vi "UI.vi"(8 "error":errorcluster, 11 "2-axis":refnum<class "Syncronus 2-Axis Stage.lvclass">) -> (0 "error out":errorcluster)   [LabVIEW 2022 SP3, in "Controls.lvlib"]
uses:
  View/Controls.lvlib
  Syncronus 2-Axis Stage/Syncronus 2-Axis Stage.lvclass
panel:
  out "XY Position Graph":cluster{"X":dbl, "Y":dbl}[](graph)
  in  "Clear Error":bool
  in  "Set X-Speed":u16
  in  "Set Y-Speed":u16
  in  "Set X-Acceleration":u16
  in  "Set Y-Acceleration":u16
  out "X-Speed":dbl
  out "Y-Speed":dbl
  out "X-Current Speed":dbl
  out "Y-Current Speed":dbl
  out "X-Acceleration":dbl
  out "Y-Acceleration":dbl
  out "Y-Homed":bool
  out "X-Homed":bool
  out "X-Moving":bool
  out "Y-Moving":bool
  out "Y-Position":dbl
  out "X-Position":dbl
  out "Stage Error":errorcluster
  in  "Abort Motion":bool
  in  "Home Stage":bool
  in  "Move Stage":bool
  in  "Y-Destination":dbl
  in  "X-Destination":dbl
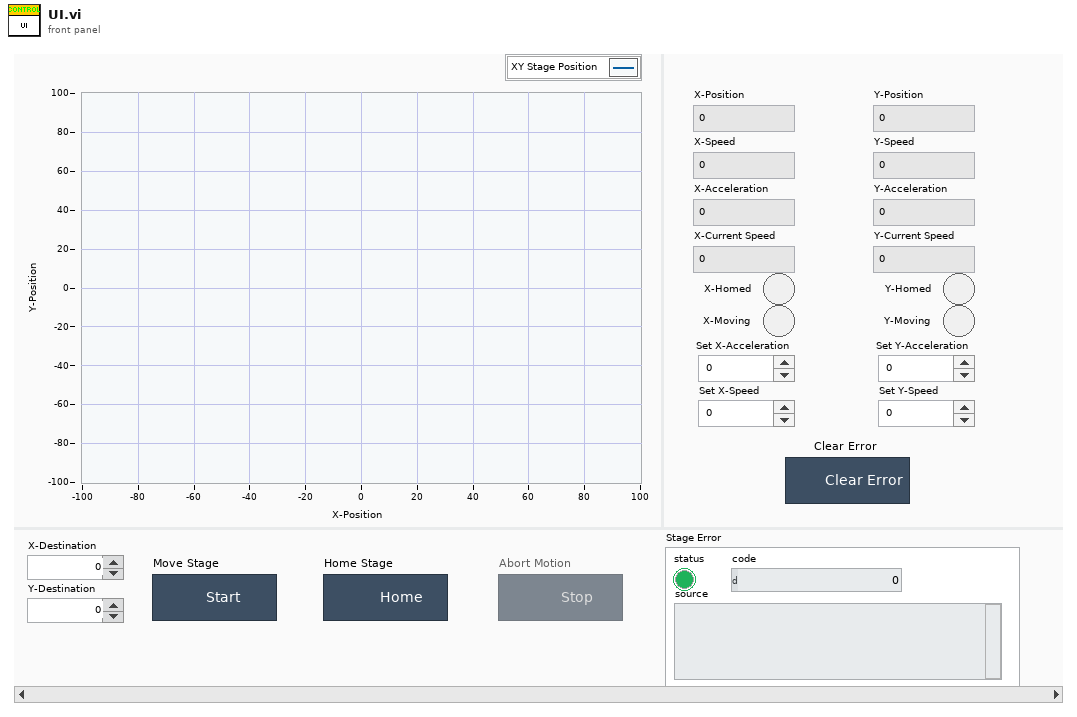
[diagram p1: front panel]
types:
  T1 = enum32{"Invalid", "Standard", "Closed", "Hidden", "Minimized", "Maximized"}
  T2 = enum32{"invalid app kind", "Development System", "Run Time System", "Student Edition", "Embedded LabVIEW", "Evaluation", "Custom"}
  T3 = enum8{"Enabled", "Disabled", "Disabled and Grayed Out"}
  T4 = cluster{"Core":cluster{"Current VI Reference":refnum<vi>, "Close Panel on Exit?":bool}, "2-axis":refnum<class "Syncronus 2-Axis Stage.lvclass">}
  T5 = cluster{"Current VI Reference":refnum<vi>, "Close Panel on Exit?":bool}
  T6 = cluster{"Current Position X":dbl, "Current Position Y":dbl}[]
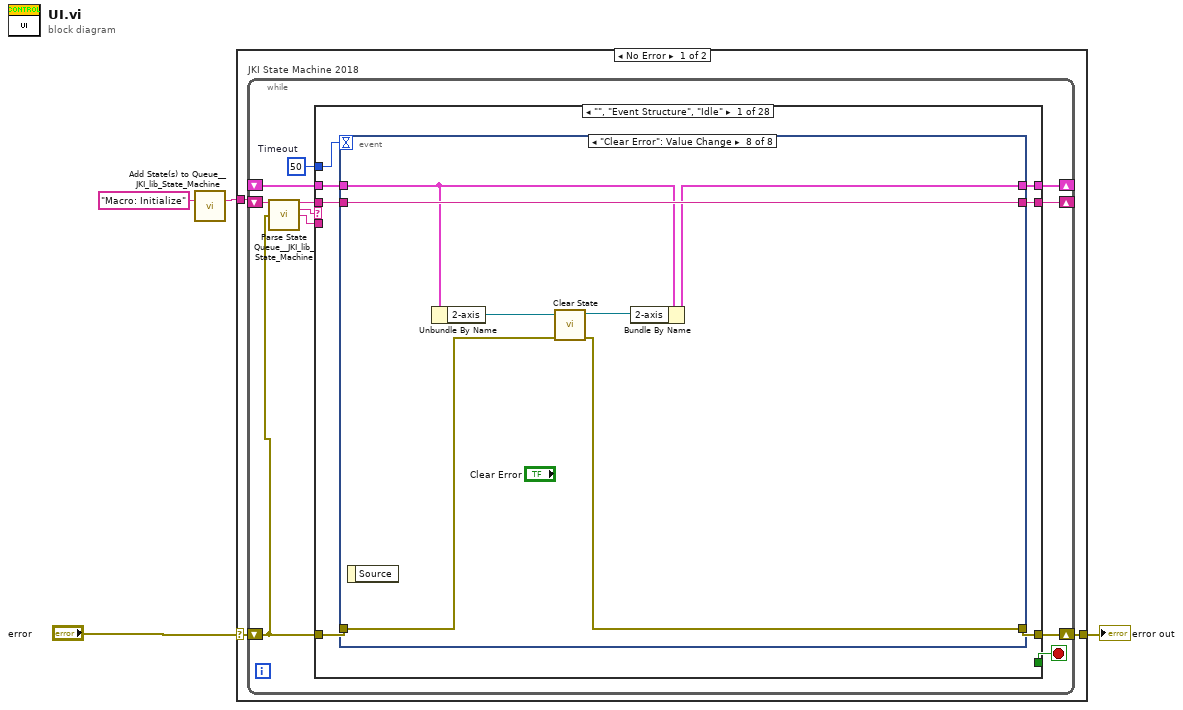
[diagram p0: block diagram]
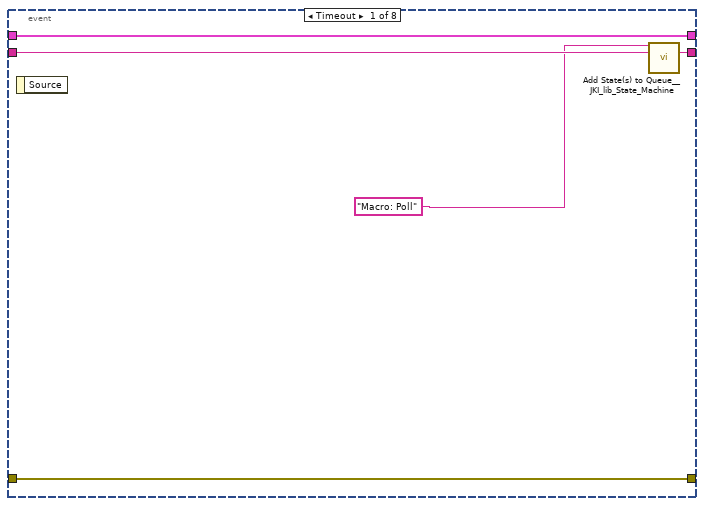
[diagram p2: hidden frame]
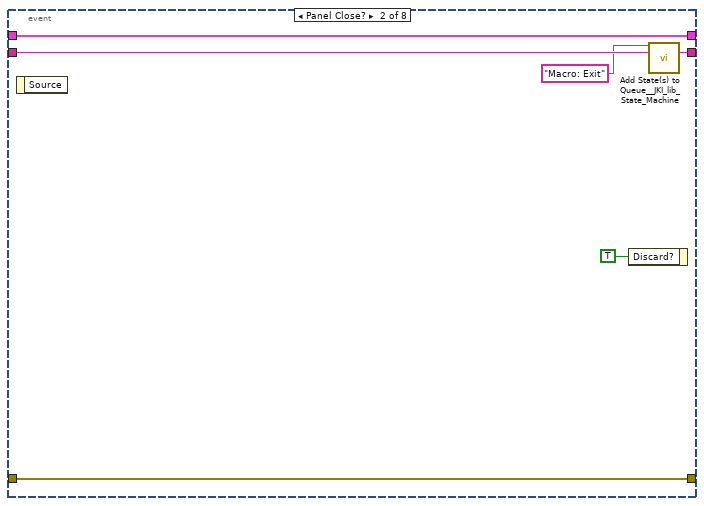
[diagram p3: hidden frame]
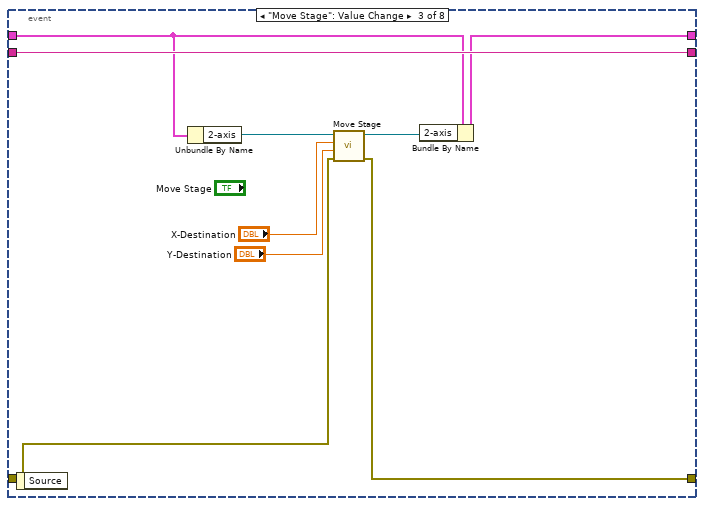
[diagram p4: hidden frame]
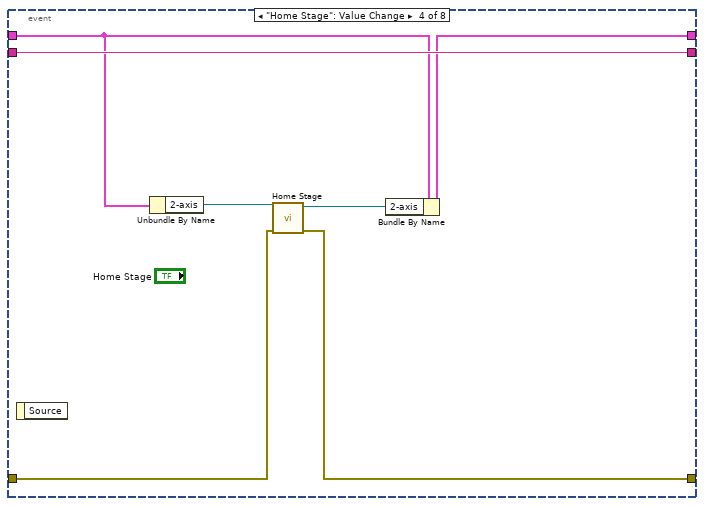
[diagram p5: hidden frame]
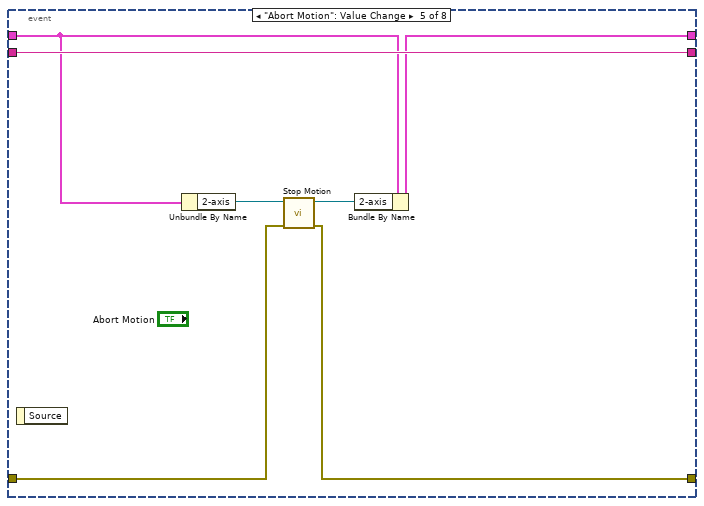
[diagram p6: hidden frame]
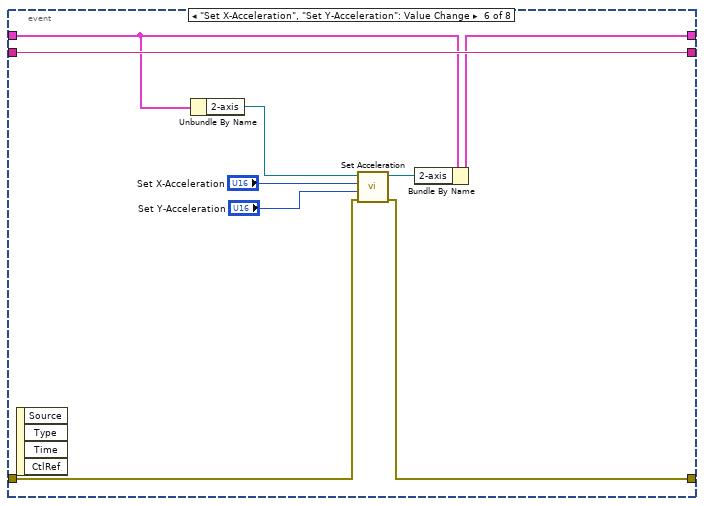
[diagram p7: hidden frame]
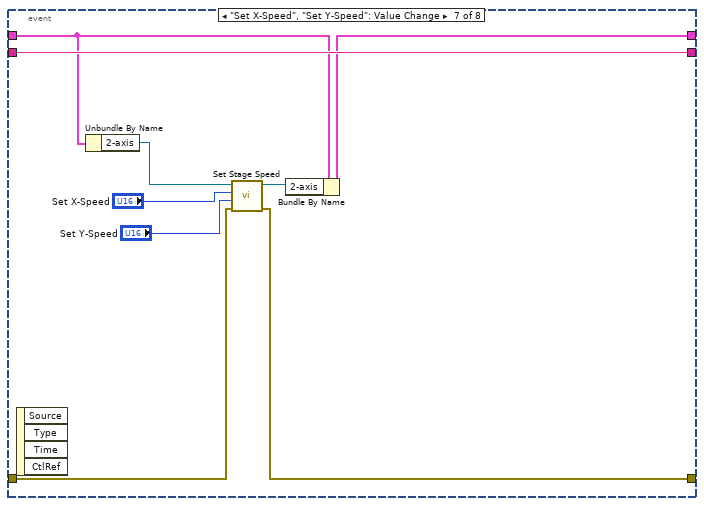
[diagram p8: hidden frame]
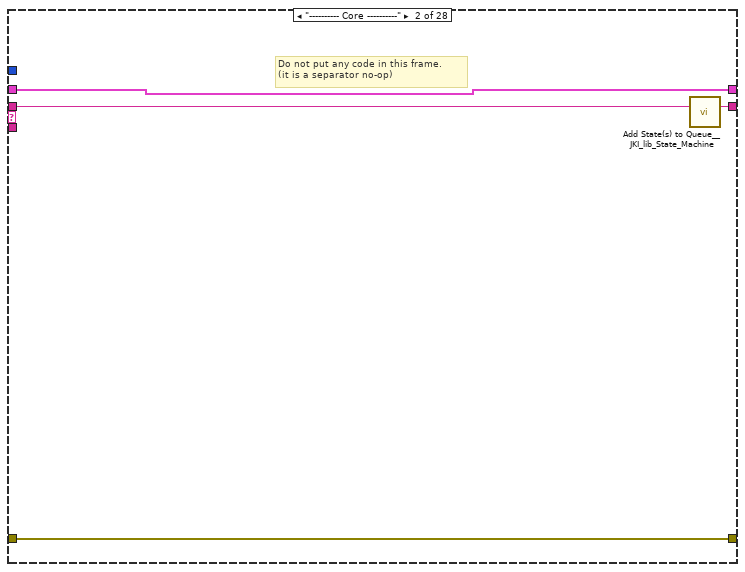
[diagram p9: hidden frame]
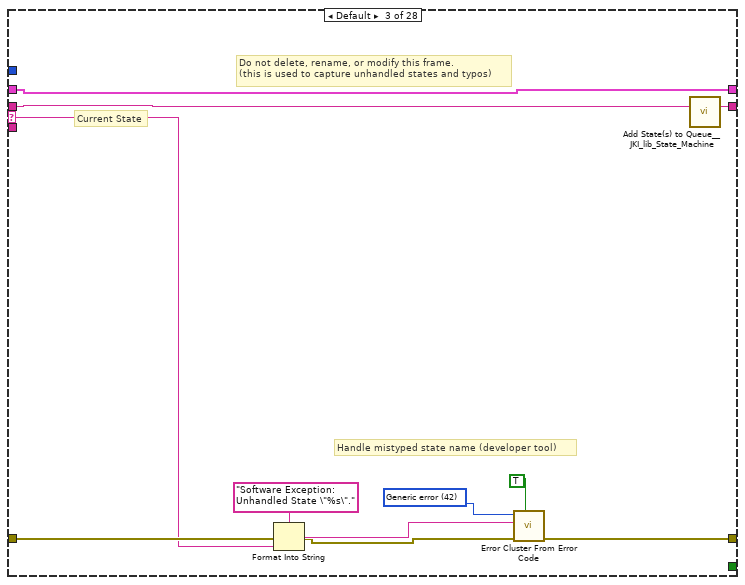
[diagram p10: hidden frame]
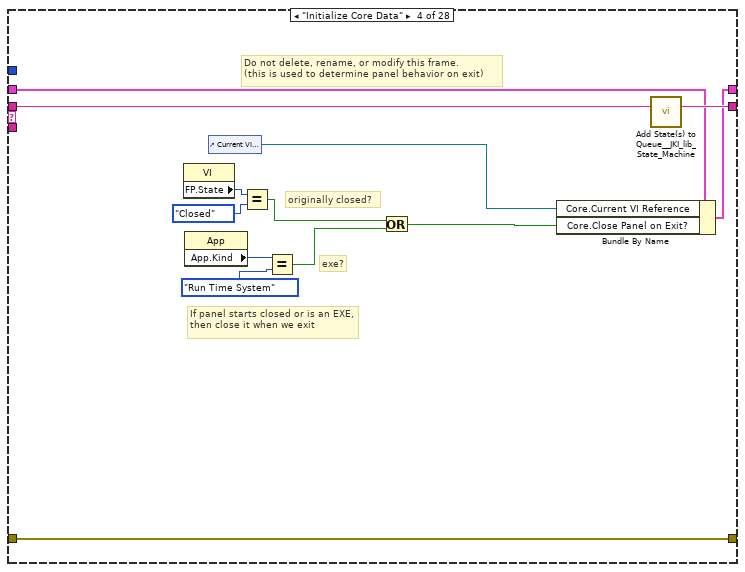
[diagram p11: hidden frame]
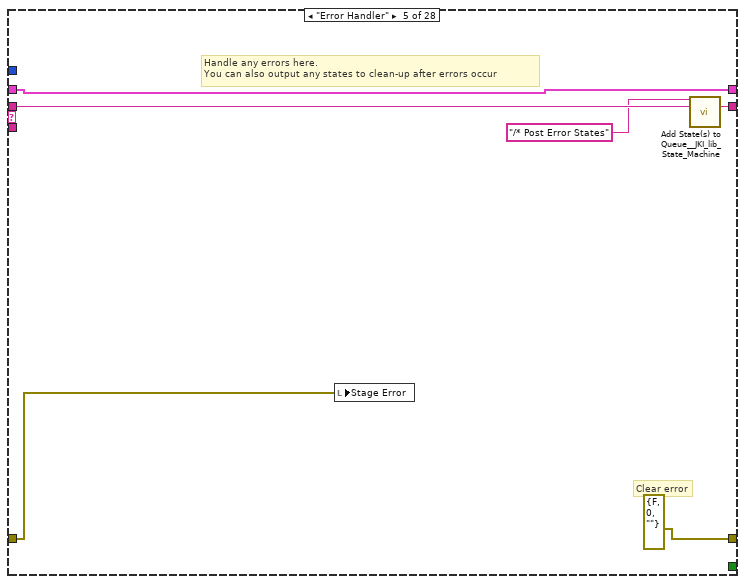
[diagram p12: hidden frame]
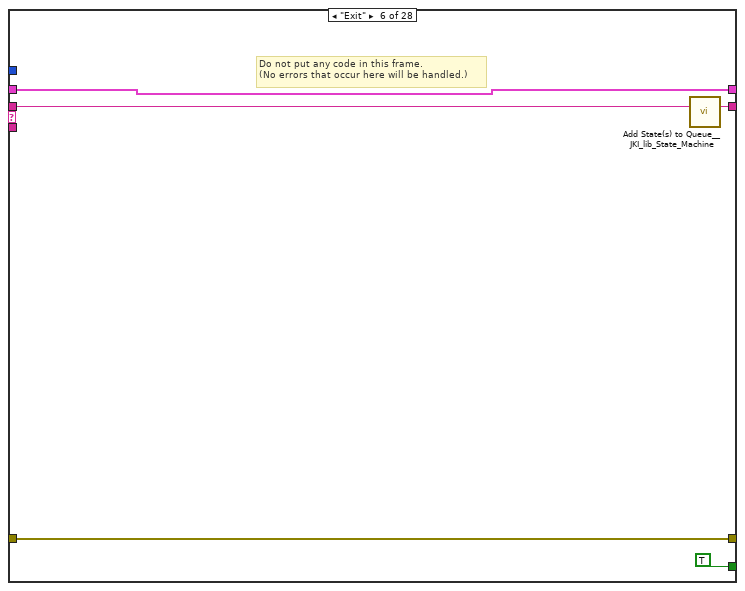
[diagram p13: hidden frame]
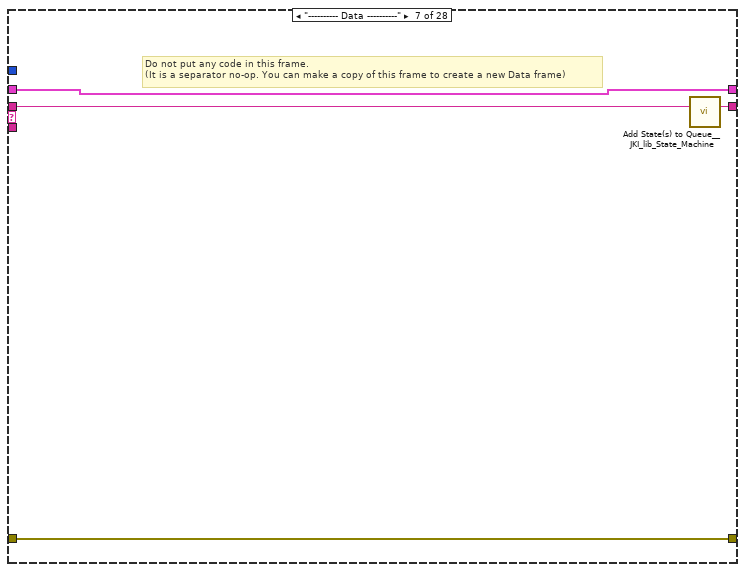
[diagram p14: hidden frame]
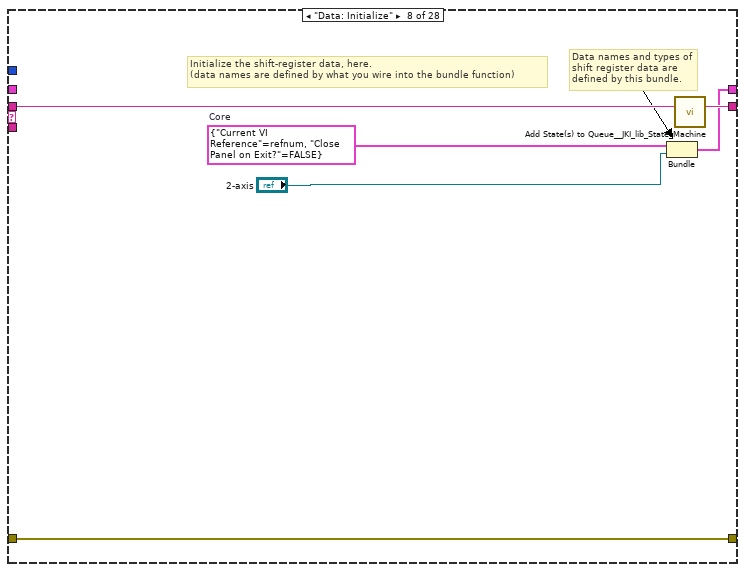
[diagram p15: hidden frame]
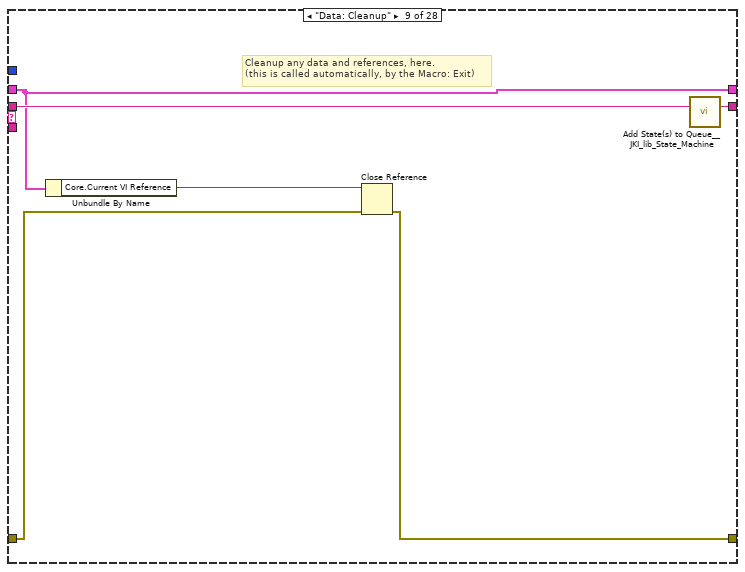
[diagram p16: hidden frame]
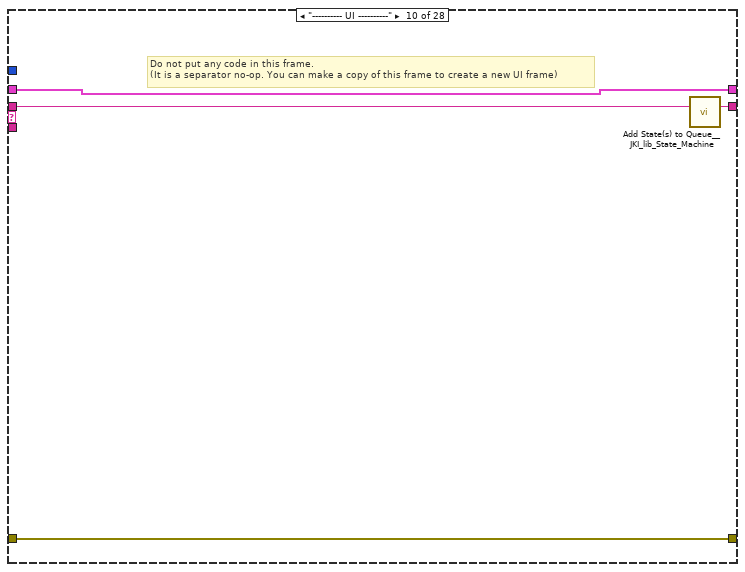
[diagram p17: hidden frame]
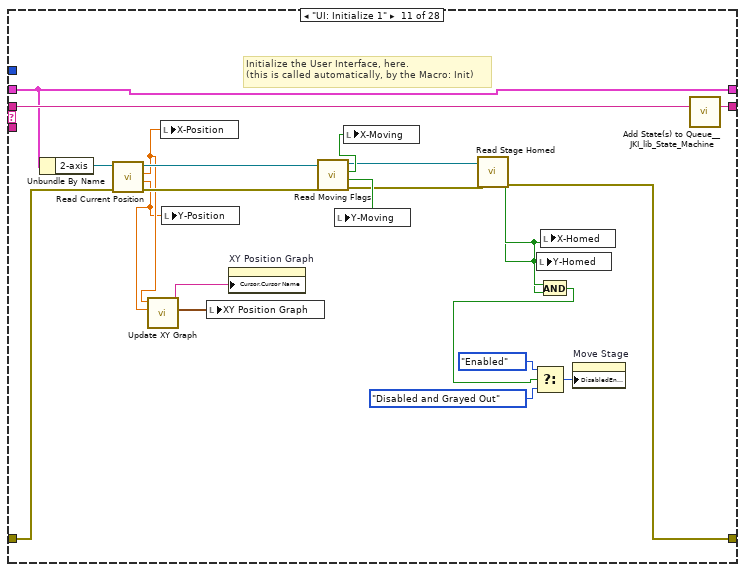
[diagram p18: hidden frame]
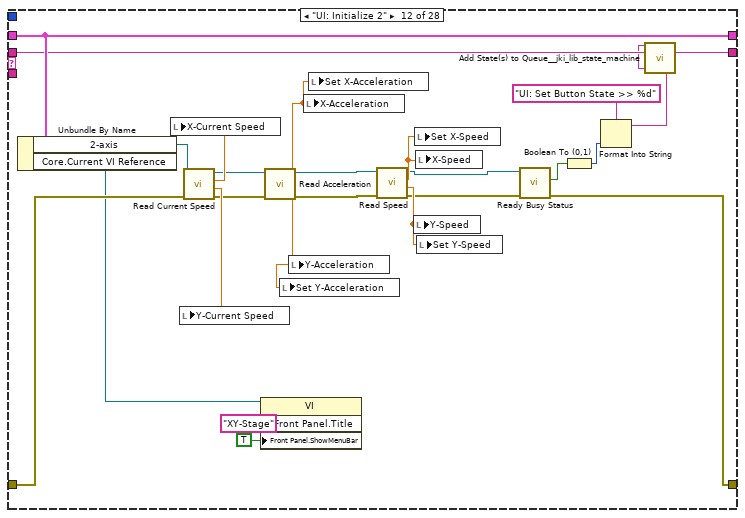
[diagram p19: hidden frame]
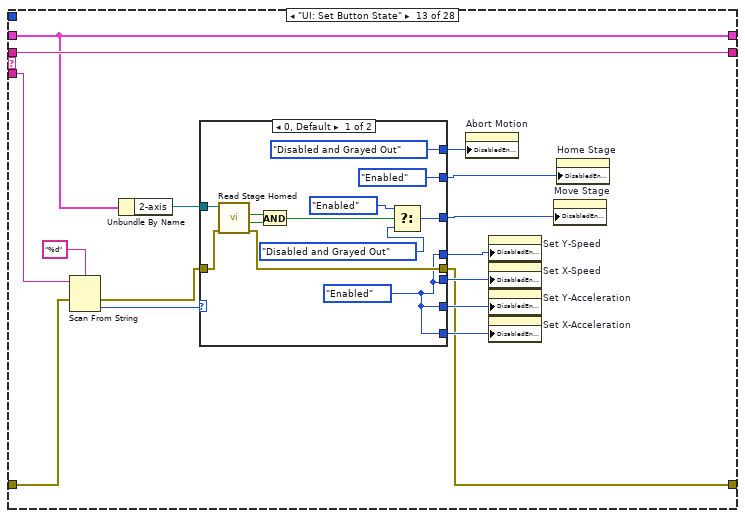
[diagram p20: hidden frame]
diagram:
  n1 = call <vilib>:"Add State(s) to Queue__JKI_lib_State_Machine.vi"("State(s) in (\"\")"="Macro: Initialize") -> ("States Out"=w1:string)  [unwired: 14 in]
  n2 = case shown="No Error" "error" {
    selector: "error" -> [w7 _]
    tunnel: [w6 _] -> w3
    tunnel: w1 -> [w5 _]
    frame No Error {
      n3 = while "JKI State Machine 2018" {
        shift-right: [w11] -> _
        shift-left: _ -> [w10]
        shift-right: [w14] -> w6
        shift-left: w7 -> [w8]
        shift-right: [w13] -> _
        shift-left: w5 -> [w15]
        stop <- w12 stop-if-true
        w9 = 50  # Timeout
        n4 = call <vilib>:"Parse State Queue__JKI_lib_State_Machine.vi"("State Queue"=w15, "Error In (no error)"=w8) -> ("Remaining States"=w17:string, "Current State"=w18:string, "Arguments"=w16:string)  [unwired: 11 in]
        n5 = case shown="\"\", \"Event Structure\", \"Idle\"" w18 {
          selector: w18 -> [_ _ w89 _ _ _ _ _ _ _ _ _ _ _ _ _ _ _ _ _ _ _ _ _ _ _ _ _]
          tunnel: w17 -> [w25 w88 w93 w112 w118 w123 w127 w133 w139 w143 w165 w177 w206 w227 w238 w307 w312 w322 w325 w330 w342 w351 w360 w369 w378 w384 w399 w407]
          tunnel: w16 -> [_ _ _ _ _ _ _ _ _ _ _ _ w196 w222 w232 _ _ _ _ _ _ _ _ _ _ _ _ _]
          tunnel: w10 -> [w23 w85 w91 w105 w115 w121 w124 _ w134 w140 w163 w180 w198 w225 w234 w304 w309 w319 w327 w329 w339 w350 w359 w368 w377 w388 w398 w406]
          tunnel: [w22 w86 w95 w109 errorcluster {"status"=FALSE, "code"=0, "source"=""} ("error out") w120 w125 w130 w135 w141 w149 w172 w193 w223 w235 w305 w310 w320 w323 w328 w333 w345 w354 w363 w372 w381 w395 w402] -> w14
          tunnel: w8 -> [w21 w86 w94 w109 w113 w120 w125 w130 w136 w141 w156 w179 w192 w224 w236 w305 w310 w320 w323 w328 w335 w346 w355 w364 w373 w382 w396 w403]
          tunnel: [w24 w87 w92 w111 w117 w122 w126 w132 w138 w142 w164 w178 w206 w226 w237 w306 w311 w321 w326 w330 w342 w351 w360 w369 w378 w385 w399 w407] -> w13
          tunnel: [_ _ _ _ _ TRUE _ _ _ _ _ _ _ _ _ _ _ _ _ _ _ _ _ _ _ _ _ _] -> w12
          tunnel: [w20 w85 w91 w110 w115 w121 w124 w131 w134 w140 w163 w180 w198 w225 w234 w304 w309 w319 w327 w329 w332 w344 w353 w362 w371 w380 w392 w401] -> w11
          tunnel: w9 -> [w19 _ _ _ _ _ _ _ _ _ _ _ _ _ _ _ _ _ _ _ _ _ _ _ _ _ _ _]
          frame "", "Event Structure", "Idle" {
            n6 = event shown="[7] \"Clear Error\": Value Change" {
              selector: _ -> [_ _ _ _ _ _ _ _]
              dyn-events: _ -> [_ _ _ _ _ _ _ _]
              timeout: w19 -> [_ _ _ _ _ _ _ _]
              tunnel: w25 -> [w30 w36 w45 w52 w59 w68 w77 w84]
              tunnel: [w29 w35 w45 w52 w59 w68 w77 w84] -> w24
              tunnel: w23 -> [w27 w33 w44 w51 w58 w67 w76 w83]
              tunnel: [w28 w34 w40 w49 w57 w63 w74 w81] -> w22
              tunnel: w21 -> [w28 w34 w41 w50 w56 w64 w75 w82]
              tunnel: [w27 w33 w38 w47 w54 w61 w70 w79] -> w20
              event Timeout {
                n7 = event-data() -> ()  [unwired: 1 in, 1 out]
                n8 = call <vilib>:"Add State(s) to Queue__JKI_lib_State_Machine.vi"("State(s) in Front (\"\")"="Macro: Poll", "State(s) in (\"\")"=w30) -> ("States Out"=w29:string)  [unwired: 13 in]
              }
              event Panel Close? {
                n9 = event-data() -> ()  [unwired: 1 in, 1 out]
                n10 = event-data("Discard?"=TRUE) -> ()  [unwired: 1 in, 1 out]
                n11 = call <vilib>:"Add State(s) to Queue__JKI_lib_State_Machine.vi"("State(s) in Front (\"\")"="Macro: Exit", "State(s) in (\"\")"=w36) -> ("States Out"=w35:string)  [unwired: 13 in]
              }
              event "Move Stage": Value Change {
                n12 = event-data() -> ()  [unwired: 1 in, 1 out]
                n13 = Unbundle By Name(w44) -> ("2-axis"=w39:refnum<class "Syncronus 2-Axis Stage.lvclass">)
                n14 = call-dynamic "Move Stage.vi"("error in (no error)"=w41, "Y Axis"="Y-Destination", "X Axis"="X-Destination", "2-Axis Stage in"=w39) -> ("error out"=w40:errorcluster, "2-Axis Stage out"=w37:refnum<class "Syncronus 2-Axis Stage.lvclass">)  [unwired: 6 in]
                n15 = Bundle By Name(cluster=w44, "2-axis"=w37) -> (w38:T4)
              }
              event "Home Stage": Value Change {
                n16 = event-data() -> ()  [unwired: 1 in, 1 out]
                n17 = Unbundle By Name(w51) -> ("2-axis"=w48:refnum<class "Syncronus 2-Axis Stage.lvclass">)
                n18 = call-dynamic "Home Stage.vi"("error in (no error)"=w50, "2-Axis Stage in"=w48) -> ("error out"=w49:errorcluster, "2-Axis Stage out"=w46:refnum<class "Syncronus 2-Axis Stage.lvclass">)  [unwired: 8 in]
                n19 = Bundle By Name(cluster=w51, "2-axis"=w46) -> (w47:T4)
              }
              event "Abort Motion": Value Change {
                n20 = event-data() -> ()  [unwired: 1 in, 1 out]
                n21 = Unbundle By Name(w58) -> ("2-axis"=w55:refnum<class "Syncronus 2-Axis Stage.lvclass">)
                n22 = call-dynamic "Stop Motion.vi"("error in (no error)"=w56, "2-Axis Stage in"=w55) -> ("error out"=w57:errorcluster, "2-Axis Stage out"=w53:refnum<class "Syncronus 2-Axis Stage.lvclass">)  [unwired: 8 in]
                n23 = Bundle By Name(cluster=w58, "2-axis"=w53) -> (w54:T4)
              }
              event "Set X-Acceleration", "Set Y-Acceleration": Value Change {
                n24 = event-data() -> ()  [unwired: 1 in, 4 out]
                n25 = Unbundle By Name(w67) -> ("2-axis"=w62:refnum<class "Syncronus 2-Axis Stage.lvclass">)
                n26 = call-dynamic "Set Acceleration.vi"("error in (no error)"=w64, "Y Axis"="Set Y-Acceleration", "X Axis"="Set X-Acceleration", "2-Axis Stage in"=w62) -> ("error out"=w63:errorcluster, "2-Axis Stage out"=w60:refnum<class "Syncronus 2-Axis Stage.lvclass">)  [unwired: 6 in]
                n27 = Bundle By Name(cluster=w67, "2-axis"=w60) -> (w61:T4)
              }
              event "Set X-Speed", "Set Y-Speed": Value Change {
                n28 = event-data() -> ()  [unwired: 1 in, 4 out]
                n29 = Unbundle By Name(w76) -> ("2-axis"=w71:refnum<class "Syncronus 2-Axis Stage.lvclass">)
                n30 = call-dynamic "Set Stage Speed.vi"("error in (no error)"=w75, "Y Axis"="Set Y-Speed", "X Axis"="Set X-Speed", "2-Axis Stage in"=w71) -> ("error out"=w74:errorcluster, "2-Axis Stage out"=w69:refnum<class "Syncronus 2-Axis Stage.lvclass">)  [unwired: 6 in]
                n31 = Bundle By Name(cluster=w76, "2-axis"=w69) -> (w70:T4)
              }
              event "Clear Error": Value Change {
                n32 = event-data() -> ()  [unwired: 1 in, 1 out]
                n33 = Unbundle By Name(w83) -> ("2-axis"=w80:refnum<class "Syncronus 2-Axis Stage.lvclass">)
                n34 = call-dynamic "Clear State.vi"("error in (no error)"=w82, "2-Axis Stage Status in"=w80) -> ("error out"=w81:errorcluster, "2-Axis Stage Status out"=w78:refnum<class "Syncronus 2-Axis Stage.lvclass">)  [unwired: 8 in]
                n35 = Bundle By Name(cluster=w83, "2-axis"=w78) -> (w79:T4)
              }
            }
          }
          frame "---------- Core ----------" {
            # "Do not put any code in this frame.\n(it is a separator no-op)"
            n36 = call <vilib>:"Add State(s) to Queue__JKI_lib_State_Machine.vi"("State(s) in (\"\")"=w88) -> ("States Out"=w87:string)  [unwired: 14 in]
          }
          frame Default {
            w98 = 42 items=["No error", "Argument error", "Memory is full", "Out of zone", "End of file", "File already open", "Generic file I/O error", "File not found", "File permission error", "Disk is full", "Duplicate path", "Too many files open", "System feature not enabled", "Resource file not found", "Cannot add resource", "Resource not found", "Image not found", "Image memory error", "Pen does not exist", "Config type invalid", "Config token not found", "Config parse error", "Config memory error", "Bad external code format", "Bad external code offset", "External code not present", "Null window", "Destroy window error", "Null menu", "Print aborted", "Bad print record", "Print driver error", "Windows error during printing", "Memory error during printing", "Print dialog error", "Generic print error", "Invalid device refnum", "Device not found", "Device parameter error", "Device unit error", "Cannot open device", "Device call aborted", "Generic error", "Cancelled by user", "Object ID too low", "Object ID too high", "Object not in heap", "Unknown heap", "Unknown object (invalid DefProc)", "Unknown object (DefProc not in table)", "Message out of range", "Invalid (null) method", "Unknown message", "Manager call not supported", "Bad address", "Network operation in progress", "Network operation timed out", "Connection is busy", "Network attribute not supported", "Network error", "Address in use", "System out of memory", "Connection aborted", "Connection refused", "Not connected", "Already connected", "Connection closed", "Initialization error (interapplication manager)", "Bad occurrence", "Wait on unbound occurrence handler", "Occurrence queue overflow", "Datalog type conflict", "Unused", "Unrecognized type (interapplication manager)", "Memory corrupt", "Failed to make temporary DLL", "Old CIN version", "Drag socket not found", "Failed to load drop-object", "Failed to register OLE object", "Failed to release OLE object", "Format specifier type mismatch", "Unknown format specifier", "Too few format specifiers", "Too many format specifiers", "Scan failed", "Newer CIN version", "Error converting to variant", "Runtime menu error", "Password tampered", "Variant attribute not found", "Incompatible variant data type", "Event data is not available", "Event Store is not present", "Occurrence is not found", "Event Queue is not created", "Event info is not available", "Refnum passed is NULL", "Error retrieving Class GUID", "Error retrieving CoClass GUID", "Error retrieving TypeLib GUID.", "Bad built application magic bytes.", "Specific driver is different from the specific driver associated with the Logical Name.", "There is no session opened to the class driver.", "Max Error", "MAX - Error with config objects", "MAX - Error loading configuration", "MAX - Group not supported"]
            # "Current State"
            # "Do not delete, rename, or modify this frame.\n(this is used to capture unhandled states and typos)"
            # "Handle mistyped state name (developer tool)"
            n37 = Format Into String(format string="Software Exception: Unhandled State \"%s\"." ("message"), error in=w94, w89) -> (resulting string=w97:string, error out=w96:errorcluster)  [unwired: 1 in]
            n38 = call <vilib>:"Error Cluster From Error Code.vi"("show call chain? (False)"=TRUE, "error in (no error)"=w96, "error message (\"\")"=w97, "error code (0)"=w98) -> ("error out"=w95:errorcluster)  [unwired: 5 in]
            n39 = call <vilib>:"Add State(s) to Queue__JKI_lib_State_Machine.vi"("State(s) in (\"\")"=w93) -> ("States Out"=w92:string)  [unwired: 14 in]
          }
          frame "Initialize Core Data" {
            # "Do not delete, rename, or modify this frame.\n(this is used to determine panel behavior on exit)"
            # "originally closed?"
            # "exe?"
            # "If panel starts closed or is an EXE, then close it when we exit"
            n40 = property class="VI"() -> ("FP.State"=w102:T1)  [unwired: 2 in, 2 out]
            n41 = property class="App"() -> ("App.Kind"=w108:T2)  [unwired: 2 in, 2 out]
            n42 = control-ref of="Current VI Reference"() -> (w103:refnum<vi>)
            n43 = Equal?(x=w102, y=T1."Closed" ("Front Panel Window:State")) -> (x = y?=w100:bool)
            n44 = Equal?(x=w108, y=T2."Run Time System" ("Application:Kind")) -> (x = y?=w106:bool)
            n45 = Or(x=w100, y=w106) -> (x .or. y?=w104:bool)
            n46 = Bundle By Name(cluster=w105, "Core.Current VI Reference"=w103, "Core.Close Panel on Exit?"=w104) -> (w110:T4)
            n47 = call <vilib>:"Add State(s) to Queue__JKI_lib_State_Machine.vi"("State(s) in (\"\")"=w112) -> ("States Out"=w111:string)  [unwired: 14 in]
          }
          frame "Error Handler" {
            # "Handle any errors here.\nYou can also output any states to clean-up after errors occur"
            # "Clear error"
            n48 = local write "Stage Error"(w113) -> ()
            n49 = call <vilib>:"Add State(s) to Queue__JKI_lib_State_Machine.vi"("State(s) in Front (\"\")"="/* Post Error States", "State(s) in (\"\")"=w118) -> ("States Out"=w117:string)  [unwired: 13 in]
          }
          frame "Exit" {
            # "Do not put any code in this frame.\n(No errors that occur here will be handled.)"
            n50 = call <vilib>:"Add State(s) to Queue__JKI_lib_State_Machine.vi"("State(s) in (\"\")"=w123) -> ("States Out"=w122:string)  [unwired: 14 in]
          }
          frame "---------- Data ----------" {
            # "Do not put any code in this frame.\n(It is a separator no-op. You can make a copy of this frame to create a new Data frame)"
            n51 = call <vilib>:"Add State(s) to Queue__JKI_lib_State_Machine.vi"("State(s) in (\"\")"=w127) -> ("States Out"=w126:string)  [unwired: 14 in]
          }
          frame "Data: Initialize" {
            w129 = T5 {"Current VI Reference"=refnum, "Close Panel on Exit?"=FALSE}  # Core
            # "Data names and types of shift register data are defined by this bundle."
            # "Initialize the shift-register data, here.\n(data names are defined by what you wire into the bundle function)"
            n52 = Bundle("Core"=w129, "2-axis"="2-axis") -> (w131:T4)  [unwired: 1 in]
            n53 = call <vilib>:"Add State(s) to Queue__JKI_lib_State_Machine.vi"("State(s) in (\"\")"=w133) -> ("States Out"=w132:string)  [unwired: 14 in]
          }
          frame "Data: Cleanup" {
            # "Cleanup any data and references, here.\n(this is called automatically, by the Macro: Exit)"
            n54 = Unbundle By Name(w134) -> ("Core.Current VI Reference"=w137:refnum<vi>)
            n55 = Close Reference(reference=w137, error in (no error)=w136) -> (error out=w135:errorcluster)
            n56 = call <vilib>:"Add State(s) to Queue__JKI_lib_State_Machine.vi"("State(s) in (\"\")"=w139) -> ("States Out"=w138:string)  [unwired: 14 in]
          }
          frame "---------- UI ----------" {
            # "Do not put any code in this frame.\n(It is a separator no-op. You can make a copy of this frame to create a new UI frame)"
            n57 = call <vilib>:"Add State(s) to Queue__JKI_lib_State_Machine.vi"("State(s) in (\"\")"=w143) -> ("States Out"=w142:string)  [unwired: 14 in]
          }
          frame "UI: Initialize 1" {
            # "Initialize the User Interface, here.\n(this is called automatically, by the Macro: Init)"
            n58 = Unbundle By Name(w163) -> ("2-axis"=w144:refnum<class "Syncronus 2-Axis Stage.lvclass">)
            n59 = call-dynamic "Read Current Position.vi"("error in (no error)"=w156, "2-Axis Stage Status in"=w144) -> ("error out"=w158:errorcluster, "Y Position"=w147:dbl, "X Position"=w148:dbl, "2-Axis Stage Status out"=w160:refnum<class "Syncronus 2-Axis Stage.lvclass">)  [unwired: 6 in]
            n60 = call "Update XY Graph.vi"("Current Position Y"=w147, "Current Position X"=w148) -> ("Array"=w146:T6, "String"=w145:string)  [unwired: 7 in, 1 out]
            n61 = local write "X-Position"(w148) -> ()
            n62 = local write "Y-Position"(w147) -> ()
            n63 = local write "XY Position Graph"(w146) -> ()
            n64 = property on="XY Position Graph" class="XYGraph (strict)"("Cursor.Cursor Name"=w145) -> ()  [unwired: 2 in, 2 out]
            n65 = call-dynamic "Read Moving Flags.vi"("error in (no error)"=w158, "2-Axis Stage Status in"=w160) -> ("error out"=w157:errorcluster, "Y-Axis Moving"=w161:bool, "X-Axis Moving"=w162:bool, "2-Axis Stage Status out"=w159:refnum<class "Syncronus 2-Axis Stage.lvclass">)  [unwired: 6 in]
            n66 = local write "Y-Moving"(w161) -> ()
            n67 = local write "X-Moving"(w162) -> ()
            n68 = call-dynamic "Read Stage Homed.vi"("error in (no error)"=w157, "2-Axis Stage Status in"=w159) -> ("error out"=w149:errorcluster, "Y-Axis Homed Moving"=w154:bool, "X-Axis Homed"=w155:bool)  [unwired: 6 in, 1 out]
            n69 = local write "Y-Homed"(w154) -> ()
            n70 = And(x=w155, y=w154) -> (x .and. y?=w153:bool)
            n71 = Select(t=T3."Enabled" ("Disabled"), s=w153, f=T3."Disabled and Grayed Out" ("Disabled")) -> (s? t:f=w151:T3)
            n72 = local write "X-Homed"(w155) -> ()
            n73 = property on="Move Stage" class="Bool"("DisabledEnum"=w151) -> ()  [unwired: 2 in, 2 out]
            n74 = call <vilib>:"Add State(s) to Queue__JKI_lib_State_Machine.vi"("State(s) in (\"\")"=w165) -> ("States Out"=w164:string)  [unwired: 14 in]
          }
          frame "UI: Initialize 2" {
            n75 = Unbundle By Name(w180) -> ("2-axis"=w166:refnum<class "Syncronus 2-Axis Stage.lvclass">, "Core.Current VI Reference"=w169:refnum<vi>)
            n76 = call-dynamic "Read Current Speed.vi"("error in (no error)"=w179, "2-Axis Stage Status in"=w166) -> ("error out"=w187:errorcluster, "Y Current Speed"=w190:dbl, "X Current Speed"=w189:dbl, "2-Axis Stage Status out"=w188:refnum<class "Syncronus 2-Axis Stage.lvclass">)  [unwired: 6 in]
            n77 = local write "X-Current Speed"(w189) -> ()
            n78 = local write "Y-Current Speed"(w190) -> ()
            n79 = property class="VI"(reference=w169, "Front Panel.Title"="XY-Stage" ("Front Panel Window:Title"), "Front Panel.ShowMenuBar"=TRUE ("Front Panel Window:Show Menu Bar")) -> ()  [unwired: 1 in, 2 out]
            n80 = call-dynamic "Read Acceleration.vi"("error in (no error)"=w187, "2-Axis Stage Status in"=w188) -> ("error out"=w185:errorcluster, "Y Acceleration"=w181:dbl, "X Acceleration"=w182:dbl, "2-Axis Stage Status out"=w186:refnum<class "Syncronus 2-Axis Stage.lvclass">)  [unwired: 6 in]
            n81 = local write "Set Y-Acceleration"(w181) -> ()
            n82 = local write "Y-Acceleration"(w181) -> ()
            n83 = local write "X-Acceleration"(w182) -> ()
            n84 = local write "Set X-Acceleration"(w182) -> ()
            n85 = call-dynamic "Read Speed.vi"("error in (no error)"=w185, "2-Axis Stage Status in"=w186) -> ("error out"=w173:errorcluster, "Y-Axis Speed"=w183:dbl, "X-Axis Speed"=w184:dbl, "2-Axis Stage Status out"=w174:refnum<class "Syncronus 2-Axis Stage.lvclass">)  [unwired: 6 in]
            n86 = local write "Y-Speed"(w183) -> ()
            n87 = local write "Set X-Speed"(w184) -> ()
            n88 = local write "X-Speed"(w184) -> ()
            n89 = local write "Set Y-Speed"(w183) -> ()
            n90 = call-dynamic "Ready Busy Status.vi"("error in (no error)"=w173, "2-Axis Stage Status in"=w174) -> ("error out"=w172:errorcluster, "Busy"=w171:bool)  [unwired: 7 in, 1 out]
            n91 = Boolean To (0,1)(Boolean=w171) -> (0, 1=w170:i16)
            n92 = Format Into String(format string="UI: Set Button State >> %d", w170) -> (resulting string=w175:string)  [unwired: 2 in, 1 out]
            n93 = call <vilib>:"Add State(s) to Queue__jki_lib_state_machine.vi"("State(s) in Front (\"\")"=w175, "State(s) in (\"\")"=w177) -> ("States Out"=w178:string)  [unwired: 13 in]
          }
          frame "UI: Set Button State" {
            n94 = Scan From String(format string="%d", input string=w196, error in=w192) -> (error out=w191:errorcluster, output 1=w194:i32)  [unwired: 2 in, 2 out]
            n95 = Unbundle By Name(w198) -> ("2-axis"=w197:refnum<class "Syncronus 2-Axis Stage.lvclass">)
            n96 = case shown="0, Default" w194 {
              tunnel: [T3."Enabled" ("Disabled") w220] -> w205
              tunnel: [T3."Disabled and Grayed Out" ("Disabled") T3."Enabled" ("Disabled")] -> w204
              tunnel: [w211 w220] -> w203
              tunnel: [w210 w219] -> w193
              tunnel: [w209 w220] -> w202
              tunnel: [w209 w220] -> w201
              tunnel: [w209 w220] -> w200
              tunnel: [w209 w220] -> w199
              tunnel: w197 -> [w207 _]
              tunnel: w191 -> [w208 w219]
              frame 0, Default {
                w209 = T3."Enabled" ("Disabled")
                n97 = call-dynamic "Read Stage Homed.vi"("error in (no error)"=w208, "2-Axis Stage Status in"=w207) -> ("error out"=w210:errorcluster, "Y-Axis Homed Moving"=w215:bool, "X-Axis Homed"=w216:bool)  [unwired: 6 in, 1 out]
                n98 = And(x=w216, y=w215) -> (x .and. y?=w214:bool)
                n99 = Select(t=T3."Enabled" ("Disabled"), s=w214, f=T3."Disabled and Grayed Out" ("Disabled")) -> (s? t:f=w211:T3)
              }
              frame 1 {
                w220 = T3."Disabled and Grayed Out" ("Disabled")
              }
            }
            n100 = property on="Abort Motion" class="Bool"("DisabledEnum"=w204) -> ()  [unwired: 2 in, 2 out]
            n101 = property on="Set Y-Speed" class="DigNum (strict)"("DisabledEnum"=w202) -> ()  [unwired: 2 in, 2 out]
            n102 = property on="Set X-Speed" class="DigNum (strict)"("DisabledEnum"=w201) -> ()  [unwired: 2 in, 2 out]
            n103 = property on="Set Y-Acceleration" class="DigNum (strict)"("DisabledEnum"=w200) -> ()  [unwired: 2 in, 2 out]
            n104 = property on="Set X-Acceleration" class="DigNum (strict)"("DisabledEnum"=w199) -> ()  [unwired: 2 in, 2 out]
            n105 = property on="Move Stage" class="Bool"("DisabledEnum"=w203) -> ()  [unwired: 2 in, 2 out]
            n106 = property on="Home Stage" class="Bool"("DisabledEnum"=w205) -> ()  [unwired: 2 in, 2 out]
          }
          frame "UI: Cursor Set" {
            # "Argument"
            # "Set and Unset Cursor Busy.\n(Usage: \"UI: Cursor Set >> Busy|Idle\")"
            n107 = case shown="\"Idle\", Default" w222 {
              tunnel: w224 -> [w229 w231]
              tunnel: [w228 w230] -> w223
              frame "Idle", Default {
                n108 = call <vilib>:"Unset Busy.vi"("error in (no error)"=w229) -> ("error out"=w228:errorcluster)  [unwired: 10 in]
              }
              frame "Busy" {
                n109 = call <vilib>:"Set Busy.vi"("error in (no error)"=w231) -> ("error out"=w230:errorcluster)  [unwired: 9 in, 1 out]
              }
            }
            n110 = call <vilib>:"Add State(s) to Queue__JKI_lib_State_Machine.vi"("State(s) in (\"\")"=w227) -> ("States Out"=w226:string)  [unwired: 14 in]
          }
          frame "UI: Front Panel State" {
            # "Argument"
            # "Set Front Panel Open or Closed\n(Usage: \"UI: Front Panel State >> Open|Close\")"
            n111 = Unbundle By Name(w234) -> ("Core.Current VI Reference"=w233:refnum<vi>)
            n112 = case shown="\"Minimize\", \"Minimized\"" w232 {
              tunnel: w236 -> [w244 w259 w270 w283 w296]
              tunnel: [w246 w260 w272 w285 w298] -> w235
              tunnel: w233 -> [w245 w257 w271 w284 w297]
              frame "Open", "Standard", Default {
                w239 = T1."Standard" ("State")
                n113 = property class="VI"(reference=w245, error in=w244) -> (reference out=w242:refnum<vi>, error out=w243:errorcluster, "FP.State"=w241:T1)
                n114 = Not Equal?(x=w241, y=w239) -> (x != y?=w240:bool)
                n115 = case shown="True" w240 {
                  tunnel: [w250 w252] -> w246
                  tunnel: w243 -> [w249 w252]
                  tunnel: w242 -> [w248 _]
                  tunnel: w239 -> [w247 _]
                  frame True {
                    n116 = invoke class="VI" method="FP.Open"(reference=w248, error in=w249, "Activate"=TRUE, "State"=w247) -> (error out=w250:errorcluster)  [unwired: 1 in, 4 out]
                  }
                  frame False {
                  }
                }
              }
              frame "Close", "Closed" {
                n117 = property class="VI"(reference=w257, error in=w259) -> (reference out=w256:refnum<vi>, error out=w258:errorcluster, "FP.State"=w254:T1)
                n118 = Not Equal?(x=w254, y=T1."Closed" ("Front Panel Window:State")) -> (x != y?=w253:bool)
                n119 = case shown="True" w253 {
                  tunnel: [w261 w264] -> w260
                  tunnel: w258 -> [w261 w263]
                  tunnel: w256 -> [_ w262]
                  frame False {
                  }
                  frame True {
                    n120 = invoke class="VI" method="FP.Close"(reference=w262, error in=w263) -> (error out=w264:errorcluster)  [unwired: 1 in, 2 out]
                  }
                }
              }
              frame "Hidden", "Hide" {
                w265 = T1."Hidden" ("State")
                n121 = property class="VI"(reference=w271, error in=w270) -> (reference out=w268:refnum<vi>, error out=w269:errorcluster, "FP.State"=w267:T1)
                n122 = Not Equal?(x=w267, y=w265) -> (x != y?=w266:bool)
                n123 = case shown="True" w266 {
                  tunnel: [w276 w277] -> w272
                  tunnel: w269 -> [w275 w277]
                  tunnel: w268 -> [w274 _]
                  tunnel: w265 -> [w273 _]
                  frame True {
                    n124 = invoke class="VI" method="FP.Open"(reference=w274, error in=w275, "State"=w273) -> (error out=w276:errorcluster)  [unwired: 2 in, 4 out]
                  }
                  frame False {
                  }
                }
              }
              frame "Minimize", "Minimized" {
                w278 = T1."Minimized" ("State")
                n125 = property class="VI"(reference=w284, error in=w283) -> (reference out=w281:refnum<vi>, error out=w282:errorcluster, "FP.State"=w280:T1)
                n126 = Not Equal?(x=w280, y=w278) -> (x != y?=w279:bool)
                n127 = case shown="True" w279 {
                  tunnel: [w289 w290] -> w285
                  tunnel: w282 -> [w288 w290]
                  tunnel: w281 -> [w287 _]
                  tunnel: w278 -> [w286 _]
                  frame True {
                    n128 = invoke class="VI" method="FP.Open"(reference=w287, error in=w288, "State"=w286) -> (error out=w289:errorcluster)  [unwired: 2 in, 4 out]
                  }
                  frame False {
                  }
                }
              }
              frame "Maximize", "Maximized" {
                w291 = T1."Maximized" ("State")
                n129 = property class="VI"(reference=w297, error in=w296) -> (reference out=w294:refnum<vi>, error out=w295:errorcluster, "FP.State"=w293:T1)
                n130 = Not Equal?(x=w293, y=w291) -> (x != y?=w292:bool)
                n131 = case shown="True" w292 {
                  tunnel: [w302 w303] -> w298
                  tunnel: w295 -> [w301 w303]
                  tunnel: w294 -> [w300 _]
                  tunnel: w291 -> [w299 _]
                  frame True {
                    n132 = invoke class="VI" method="FP.Open"(reference=w300, error in=w301, "State"=w299) -> (error out=w302:errorcluster)  [unwired: 2 in, 4 out]
                  }
                  frame False {
                  }
                }
              }
            }
            n133 = call <vilib>:"Add State(s) to Queue__JKI_lib_State_Machine.vi"("State(s) in (\"\")"=w238) -> ("States Out"=w237:string)  [unwired: 14 in]
          }
          frame "---------- Macro ----------" {
            # "Do not put any code in this frame.\n(It is a separator no-op. You can make a copy of this frame to create a new Macro frame)"
            n134 = call <vilib>:"Add State(s) to Queue__JKI_lib_State_Machine.vi"("State(s) in (\"\")"=w307) -> ("States Out"=w306:string)  [unwired: 14 in]
          }
          frame "Macro: Initialize" {
            w308 = "Data: Initialize\nInitialize Core Data\nUI: Initialize 1\nUI: Initialize 2\nUI: Front Panel State >> Open"  # Data: Initialize Initialize Core Data UI: Initialize 1 UI: Initialize 2 UI: Front Panel State >> Open
            # "Initialization Macro\n(This is called once, when the VI starts)"
            n135 = call <vilib>:"Add State(s) to Queue__JKI_lib_State_Machine.vi"("State(s) in Front (\"\")"=w308, "State(s) in (\"\")"=w312) -> ("States Out"=w311:string)  [unwired: 13 in]
          }
          frame "Macro: Exit" {
            # "Exit Macro\n(This is called once, when the VI exits)"
            n136 = Unbundle By Name(w319) -> ("Core.Close Panel on Exit?"=w318:bool)
            n137 = Select(t="UI: Front Panel State >> Close", s=w318, f="") -> (s? t:f=w315:string)
            n138 = call <vilib>:"Add State(s) to Queue__JKI_lib_State_Machine.vi"("State(s) in (\"\")"=w315, "State(s) at Back (\"\")"="Data: Cleanup\nExit") -> ("States Out"=w313:string)  [unwired: 13 in]
            n139 = call <vilib>:"Add State(s) to Queue__JKI_lib_State_Machine.vi"("State(s) in Front (\"\")"=w313, "State(s) in (\"\")"=w322) -> ("States Out"=w321:string)  [unwired: 13 in]
          }
          frame "Macro: Poll" {
            n140 = call <vilib>:"Add State(s) to Queue__jki_lib_state_machine.vi"("State(s) in Front (\"\")"="Stage: Get Latest Position\nStage: Get Moving Status\nStage: Get Homed Status\nStage: Get Acceleration\nStage: Get Current Speed\nStage: Get Busy Status\nStage: Get Speed\nStage: Get Error", "State(s) in (\"\")"=w325) -> ("States Out"=w326:string)  [unwired: 13 in]
          }
          frame "------Stage------" {
          }
          frame "Stage: Get Latest Position" {
            n141 = Unbundle By Name(w339) -> ("2-axis"=w338:refnum<class "Syncronus 2-Axis Stage.lvclass">)
            n142 = call-dynamic "Read Current Position.vi"("error in (no error)"=w335, "2-Axis Stage Status in"=w338) -> ("error out"=w334:errorcluster, "Y Position"=w336:dbl, "X Position"=w337:dbl, "2-Axis Stage Status out"=w331:refnum<class "Syncronus 2-Axis Stage.lvclass">)  [unwired: 6 in]
            "Y-Position" <- w336
            "X-Position" <- w337
            n143 = call "Update XY Graph.vi"("error in (no error)"=w334, "Current Position Y"=w336, "Current Position X"=w337) -> ("error out"=w333:errorcluster, "Array"=→"XY Position Graph":T6, "String"=w340:string)  [unwired: 6 in]
            n144 = property on="XY Position Graph" class="XYGraph (strict)"("Cursor.Cursor Name"=w340) -> ()  [unwired: 2 in, 2 out]
            n145 = Bundle By Name(cluster=w339, "2-axis"=w331) -> (w332:T4)
          }
          frame "Stage: Get Moving Status" {
            n146 = Unbundle By Name(w350) -> ("2-axis"=w349:refnum<class "Syncronus 2-Axis Stage.lvclass">)
            n147 = call-dynamic "Read Moving Flags.vi"("error in (no error)"=w346, "2-Axis Stage Status in"=w349) -> ("error out"=w345:errorcluster, "Y-Axis Moving"=→"Y-Moving":bool, "X-Axis Moving"=→"X-Moving":bool, "2-Axis Stage Status out"=w343:refnum<class "Syncronus 2-Axis Stage.lvclass">)  [unwired: 6 in]
            n148 = Bundle By Name(cluster=w350, "2-axis"=w343) -> (w344:T4)
          }
          frame "Stage: Get Homed Status" {
            n149 = Unbundle By Name(w359) -> ("2-axis"=w358:refnum<class "Syncronus 2-Axis Stage.lvclass">)
            n150 = call-dynamic "Read Stage Homed.vi"("error in (no error)"=w355, "2-Axis Stage Status in"=w358) -> ("error out"=w354:errorcluster, "Y-Axis Homed Moving"=→"Y-Homed":bool, "X-Axis Homed"=→"X-Homed":bool, "2-Axis Stage Status out"=w352:refnum<class "Syncronus 2-Axis Stage.lvclass">)  [unwired: 6 in]
            n151 = Bundle By Name(cluster=w359, "2-axis"=w352) -> (w353:T4)
          }
          frame "Stage: Get Acceleration" {
            n152 = Unbundle By Name(w368) -> ("2-axis"=w367:refnum<class "Syncronus 2-Axis Stage.lvclass">)
            n153 = call-dynamic "Read Acceleration.vi"("error in (no error)"=w364, "2-Axis Stage Status in"=w367) -> ("error out"=w363:errorcluster, "Y Acceleration"=→"Y-Acceleration":dbl, "X Acceleration"=→"X-Acceleration":dbl, "2-Axis Stage Status out"=w361:refnum<class "Syncronus 2-Axis Stage.lvclass">)  [unwired: 6 in]
            n154 = Bundle By Name(cluster=w368, "2-axis"=w361) -> (w362:T4)
          }
          frame "Stage: Get Current Speed" {
            n155 = Unbundle By Name(w377) -> ("2-axis"=w376:refnum<class "Syncronus 2-Axis Stage.lvclass">)
            n156 = call-dynamic "Read Current Speed.vi"("error in (no error)"=w373, "2-Axis Stage Status in"=w376) -> ("error out"=w372:errorcluster, "Y Current Speed"=→"Y-Current Speed":dbl, "X Current Speed"=→"X-Current Speed":dbl, "2-Axis Stage Status out"=w370:refnum<class "Syncronus 2-Axis Stage.lvclass">)  [unwired: 6 in]
            n157 = Bundle By Name(cluster=w377, "2-axis"=w370) -> (w371:T4)
          }
          frame "Stage: Get Busy Status" {
            n158 = Unbundle By Name(w388) -> ("2-axis"=w387:refnum<class "Syncronus 2-Axis Stage.lvclass">)
            n159 = call-dynamic "Ready Busy Status.vi"("error in (no error)"=w382, "2-Axis Stage Status in"=w387) -> ("error out"=w381:errorcluster, "Busy"=w386:bool, "2-Axis Stage Status out"=w379:refnum<class "Syncronus 2-Axis Stage.lvclass">)  [unwired: 7 in]
            n160 = Bundle By Name(cluster=w388, "2-axis"=w379) -> (w380:T4)
            n161 = Select(t="UI: Set Button State >>1", s=w386, f="UI: Set Button State >>0") -> (s? t:f=w383:string)
            n162 = call <vilib>:"Add State(s) to Queue__jki_lib_state_machine.vi"("State(s) in Front (\"\")"=w383, "State(s) in (\"\")"=w384) -> ("States Out"=w385:string)  [unwired: 13 in]
          }
          frame "Stage: Get Speed" {
            n163 = Unbundle By Name(w398) -> ("2-axis"=w397:refnum<class "Syncronus 2-Axis Stage.lvclass">)
            n164 = call-dynamic "Read Speed.vi"("error in (no error)"=w396, "2-Axis Stage Status in"=w397) -> ("error out"=w395:errorcluster, "Y-Axis Speed"=→"Y-Speed":dbl, "X-Axis Speed"=→"X-Speed":dbl, "2-Axis Stage Status out"=w391:refnum<class "Syncronus 2-Axis Stage.lvclass">)  [unwired: 6 in]
            n165 = Bundle By Name(cluster=w398, "2-axis"=w391) -> (w392:T4)
          }
          frame "Stage: Get Error" {
            n166 = Unbundle By Name(w406) -> ("2-axis"=w405:refnum<class "Syncronus 2-Axis Stage.lvclass">)
            n167 = call-dynamic "Read Error.vi"("error in (no error)"=w403, "2-Axis Stage Status in"=w405) -> ("error out"=w402:errorcluster, "Stage Error"=→"Stage Error":errorcluster, "2-Axis Stage Status out"=w400:refnum<class "Syncronus 2-Axis Stage.lvclass">)  [unwired: 7 in]
            n168 = Bundle By Name(cluster=w406, "2-axis"=w400) -> (w401:T4)
          }
        }
      }
    }
    frame Error {
    }
  }
  "error out" <- w3
